vi "GDSString_SetTextStyle.vi"(0 "TextIn":refnum<vi>, 1 "Start":i32[](array[numeric]), 2 "Length":i32[](array[numeric]), 3 "Style":T1(ring), 4 "Color":u32(colorbox), 5 "error in":errorcluster, 7 "Size":i32, 9 "FontName":string, 11 "PrefixAdjustment":i32) -> (14 "TextOut":refnum<vi>, 19 "error out":errorcluster)   [LabVIEW 2020]
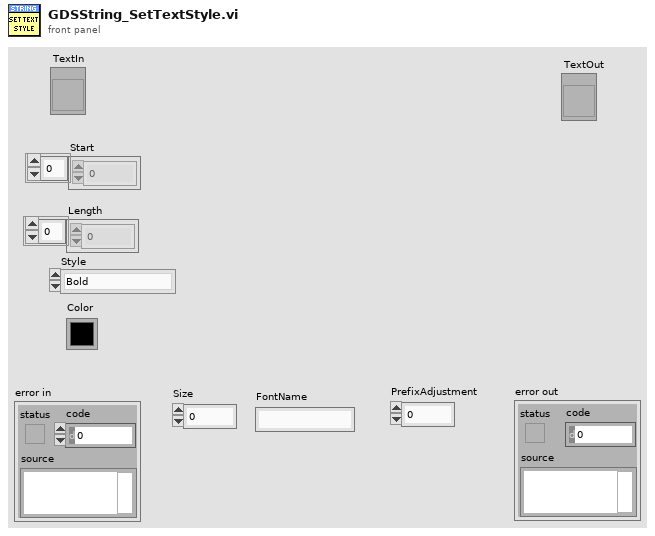
[diagram p1: front panel]
types:
  T1 = enum16{"Bold", "Italic", "StrikOut", "UnderLine", "Color", "FontSize", "FontName"}
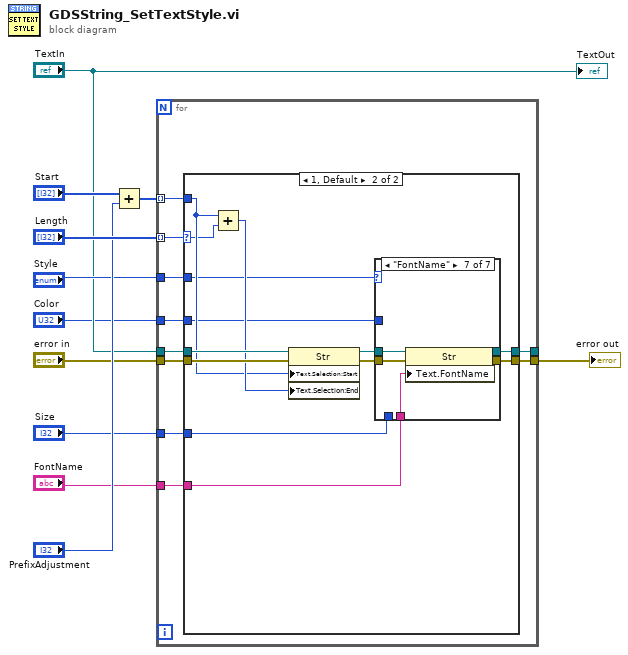
[diagram p0: block diagram]
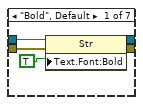
[diagram p3: hidden frame]
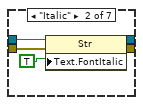
[diagram p4: hidden frame]
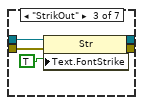
[diagram p5: hidden frame]
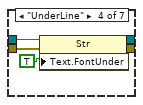
[diagram p6: hidden frame]
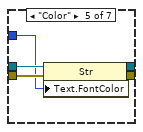
[diagram p7: hidden frame]
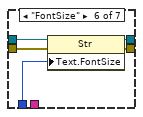
[diagram p8: hidden frame]
diagram:
  n1 = Add(x="Start", y="PrefixAdjustment") -> (x+y=w8:i32[])
  n2 = for {
    tunnel: "TextIn" -> [w21]
    tunnel: "error in" -> [w20]
    tunnel: [w19] -> w9
    tunnel: w8 -> [w18] mode=indexing
    tunnel: "Length" -> [w16] mode=indexing
    tunnel: [w17] -> _
    tunnel: "Style" -> [w15]
    tunnel: "Color" -> [w14]
    tunnel: "Size" -> [w13]
    tunnel: "FontName" -> [w12]
    n3 = case shown="1, Default" w16 {
      selector: w16 -> [_ w32]
      tunnel: w21 -> [w23 w36]
      tunnel: w20 -> [w22 w35]
      tunnel: [w22 w28] -> w19
      tunnel: w18 -> [_ w33]
      tunnel: [w23 w29] -> w17
      tunnel: w15 -> [_ w27]
      tunnel: w14 -> [_ w26]
      tunnel: w13 -> [_ w25]
      tunnel: w12 -> [_ w24]
      frame 0 {
      }
      frame 1, Default {
        n4 = Add(x=w33, y=w32) -> (x+y=w34:i32)
        n5 = property on="Property Node" class="Str"(reference=w36, error in=w35, "Text.Selection:Start"=w33, "Text.Selection:End"=w34) -> (reference out=w31:refnum<vi>, error out=w30:errorcluster)
        n6 = case shown="\"FontName\"" w27 {
          tunnel: w31 -> [w41 w46 w51 w56 w61 w66 w71]
          tunnel: w30 -> [w40 w45 w50 w55 w60 w65 w70]
          tunnel: [w39 w44 w49 w54 w59 w64 w69] -> w29
          tunnel: [w38 w43 w48 w53 w58 w63 w68] -> w28
          tunnel: w26 -> [_ _ _ _ w57 _ _]
          tunnel: w25 -> [_ _ _ _ _ w62 _]
          tunnel: w24 -> [_ _ _ _ _ _ w67]
          frame "Bold", Default {
            n7 = property on="Property Node" class="Str"(reference=w41, error in=w40, "Text.Font:Bold"=TRUE) -> (reference out=w39:refnum<vi>, error out=w38:errorcluster)
          }
          frame "Italic" {
            n8 = property on="Property Node" class="Str"(reference=w46, error in=w45, "Text.FontItalic"=TRUE ("Text.Font:Bold")) -> (reference out=w44:refnum<vi>, error out=w43:errorcluster)
          }
          frame "StrikOut" {
            n9 = property on="Property Node" class="Str"(reference=w51, error in=w50, "Text.FontStrike"=TRUE ("Text.Font:Bold")) -> (reference out=w49:refnum<vi>, error out=w48:errorcluster)
          }
          frame "UnderLine" {
            n10 = property on="Property Node" class="Str"(reference=w56, error in=w55, "Text.FontUnder"=TRUE ("Text.Font:Bold")) -> (reference out=w54:refnum<vi>, error out=w53:errorcluster)
          }
          frame "Color" {
            n11 = property on="Property Node" class="Str"(reference=w61, error in=w60, "Text.FontColor"=w57) -> (reference out=w59:refnum<vi>, error out=w58:errorcluster)
          }
          frame "FontSize" {
            n12 = property on="Property Node" class="Str"(reference=w66, error in=w65, "Text.FontSize"=w62) -> (reference out=w64:refnum<vi>, error out=w63:errorcluster)
          }
          frame "FontName" {
            n13 = property on="Property Node" class="Str"(reference=w71, error in=w70, "Text.FontName"=w67) -> (reference out=w69:refnum<vi>, error out=w68:errorcluster)
          }
        }
      }
    }
  }
  "error out" <- w9
  "TextOut" <- "TextIn"
